vi "PH_Sequencer_Watch.ProcCases.vi"(0 "i ref in":refnum<vi>, 1 "selector":string, 2 "Data":T1, 3 "call cluster":T2={"Object"="", "Selector"="", "CallType"=enum."synchronous", "Async Object"="", "Async Selector"="", "Data Descriptor"="", "Data"=[], "Error #"=0, "Expire"=0}, 5 "error in (no error)":errorcluster) -> (14 "i ref out":refnum<vi>, 17 "answer cluster":T2={"Object"="", "Selector"="", "CallType"=enum."synchronous", "Async Object"="", "Async Selector"="", "Data Descriptor"="", "Data"=[], "Error #"=0, "Expire"=0}, 19 "error out":errorcluster)   [LabVIEW 2014, in "PH_Sequencer_Watch.lvlib"]
doc: "This method is called by a process from within the default case in the event loop. The methods of a class that are linked to events will be called from THIS method. Add your code here."
uses:
  PH_Sequencer_Watch.lvlib
  CSCore/CSSystem/CoreDefs/CoreDefs.call_type.ctl
  CSCore/BaseProcess/BaseProcess.descriptor string definition.ctl
  CSCore/CSSystem/CoreDefs/CoreDefs.rawDataType.ctl
  PH_PP_Common/PH_PP_Common.PUs.ctl
  CSCore/CSSystem/CoreLib/CoreLib.string 2 byte array.vi
  CSCore/BaseProcess/BaseProcess.lvlib
  CSCore/CAEObj/CAEObj.lvlib
  CSCore/CSSystem/CoreLib/CoreLib.lvlib
  PH_Common/PH_Common.lvlib
  lib.lib/DimLVEvent/LVDimInterface/LVDimInterface.lvlib
  PH_StatusHandler/PH_StatusHandler.lvlib
  PH_BeamlineInformation/PH_BeamlineInformation.lvlib
  PH_SystemInformation/PH_SystemInformation.lvlib
  PH_PP_Common/PH_PP_Common.lvlib
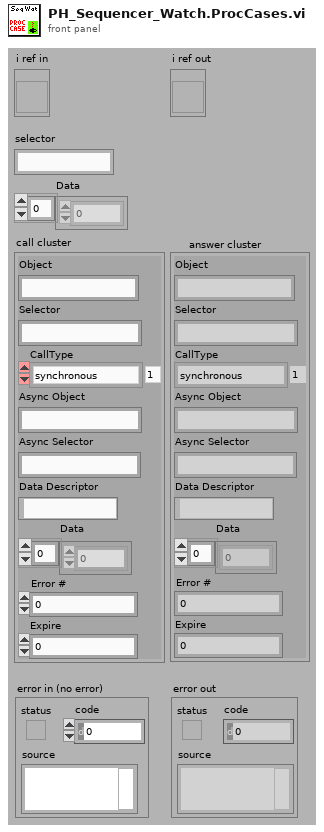
[diagram p1: front panel]
types:
  T1 = typedef "CoreDefs.rawDataType.ctl" = i8[]
  T2 = typedef "CoreDefs.call_type.ctl" = cluster{"Object":string, "Selector":string, "CallType":enum16{"simple", "synchronous", "asynchronous"}, "Async Object":string, "Async Selector":string, "Data Descriptor":T3, "Data":T1, "Error #":i32, "Expire":u32}
  T3 = typedef "BaseProcess.lvlib/BaseProcess.descriptor string definition.ctl" = string
  T4 = typedef "PH_Sequencer_Watch.lvlib/PH_Sequencer_Watch.i attribute.ctl" = cluster{"GUI Refs":cluster{"Shot ID":refnum<vi>, "Sequencer SM State":refnum<vi>, "Remaining Time":refnum<vi>, "PHELIX_Timing_T2":refnum<vi>, "T2-Unit-Dummy":refnum<vi>, "fs_Synchrolock_Watch":refnum<vi>, "Experiment_Vacuum_Control_Experiment":refnum<vi>}, "Status Synchrolock":T5, "Exp - Pressure":dbl, "Exp - Limit":dbl, "Heads":T6[], "Refs BooleanState":refnum<vi>[]}
  T5 = typedef "PH_StatusHandler.lvlib/PH_StatusHandler.Status.ctl" = i16
  T6 = typedef "PH_Sequencer_Watch.lvlib/PH_Sequencer_Watch.Head Information.ctl" = cluster{"Ref Volt":refnum<vi>, "PU":T7}
  T7 = typedef "PH_PP_Common.lvlib/PH_PP_Common.PUs.ctl" = enum16{"no Info", "PA-19mm-1", "PA-19mm-2", "PA-45mm-PILC", "PA-45mm-MAIN", "MA-PU-1", "MA-PU-2", "MA-PU-3", "MA-PU-4", "MA-PU-5", "MA-PU-6", "MA-FR", "MA-PILC", "PA-45mm-DP"}
  T8 = typedef "PH_BeamlineInformation.lvlib/PH_BeamlineInformation.i attribute.ctl" = cluster{"BL GUI Elements of Services":cluster{"Service Name":string, "GUI Elements":refnum<vi>[], "Status":i32}[], "Powermeters":T9, "Efficiency":T10, "Heads":T11[]}
  T9 = typedef "PH_BeamlineInformation.lvlib/PH_BeamlineInformation.Powermeter.ctl" = cluster{"ns FE":cluster{"GUI Ref":refnum<vi>, "Value":dbl}, "fs FE":cluster{"GUI Ref":refnum<vi>, "Value":dbl}, "PA":cluster{"GUI Ref":refnum<vi>, "Value":dbl}, "MA":cluster{"GUI Ref":refnum<vi>, "Value":dbl}, "Z6 green":cluster{"GUI Ref":refnum<vi>, "Value":dbl}, "Z6 IR":cluster{"GUI Ref":refnum<vi>, "Value":dbl}, "Z6 COS":cluster{"GUI Ref":refnum<vi>, "Value":dbl}}
  T10 = typedef "PH_BeamlineInformation.lvlib/PH_BeamlineInformation.Efficiency.ctl" = cluster{"PA Gain":cluster{"GUI Ref":refnum<vi>, "Value":dbl}, "MA Gain":cluster{"GUI Ref":refnum<vi>, "Value":dbl}, "Z6 green Conversion":cluster{"GUI Ref":refnum<vi>, "Value":dbl}, "Z6 Comp Losses":cluster{"GUI Ref":refnum<vi>, "Value":dbl}}
  T11 = typedef "PH_BeamlineInformation.lvlib/PH_BeamlineInformation.Head.ctl" = cluster{"PowerUnit":T7, "in use":cluster{"Value":bool, "GUI Ref":refnum<vi>, "linked":bool}, "voltage":cluster{"Value":dbl, "GUI Ref":refnum<vi>, "linked":bool}}
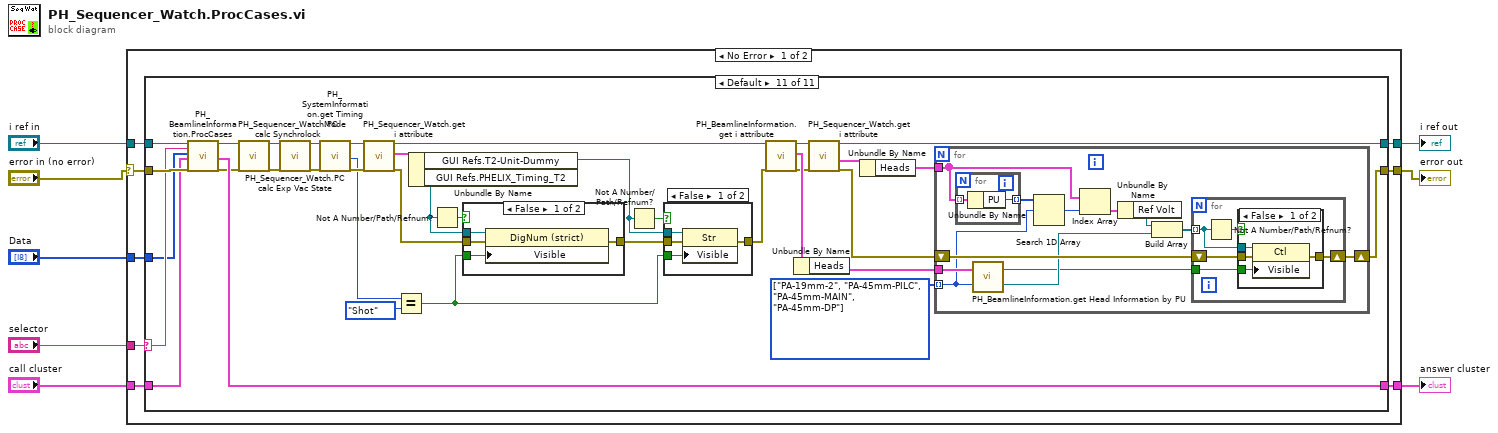
[diagram p0: block diagram]
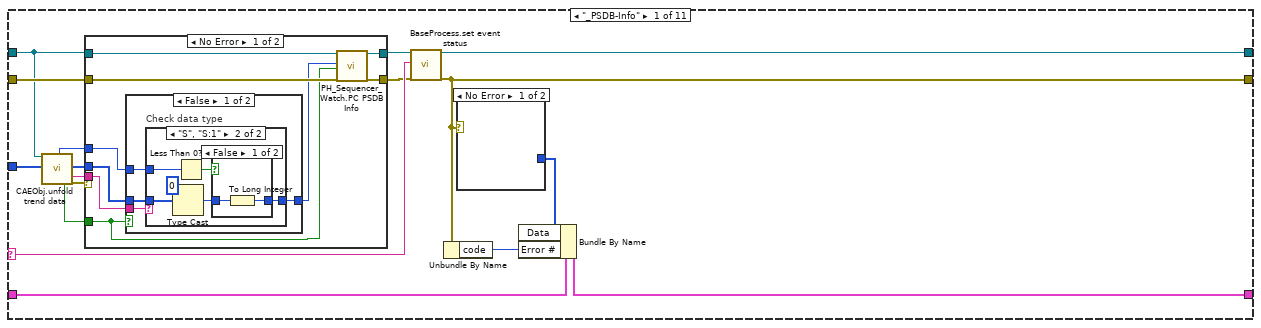
[diagram p2: hidden frame]
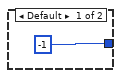
[diagram p3: hidden frame]
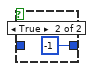
[diagram p4: hidden frame]
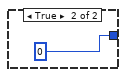
[diagram p5: hidden frame]
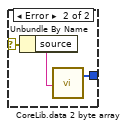
[diagram p7: hidden frame]
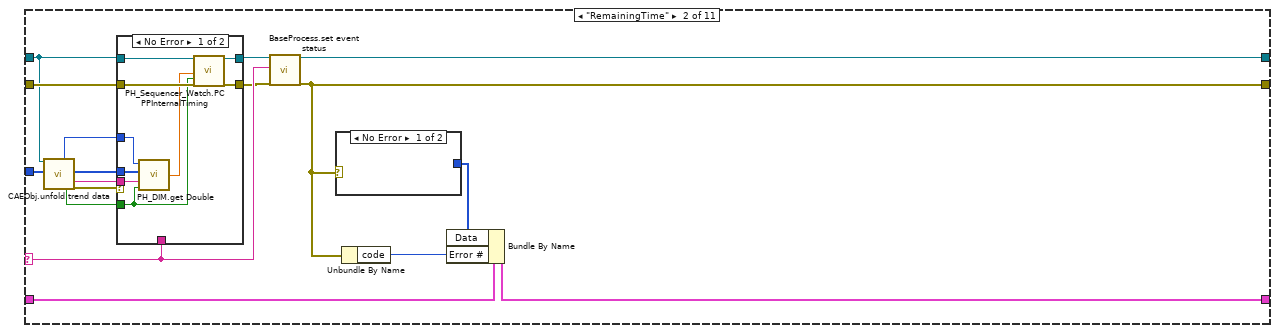
[diagram p8: hidden frame]
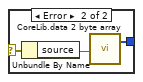
[diagram p9: hidden frame]
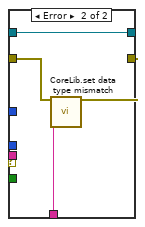
[diagram p10: hidden frame]
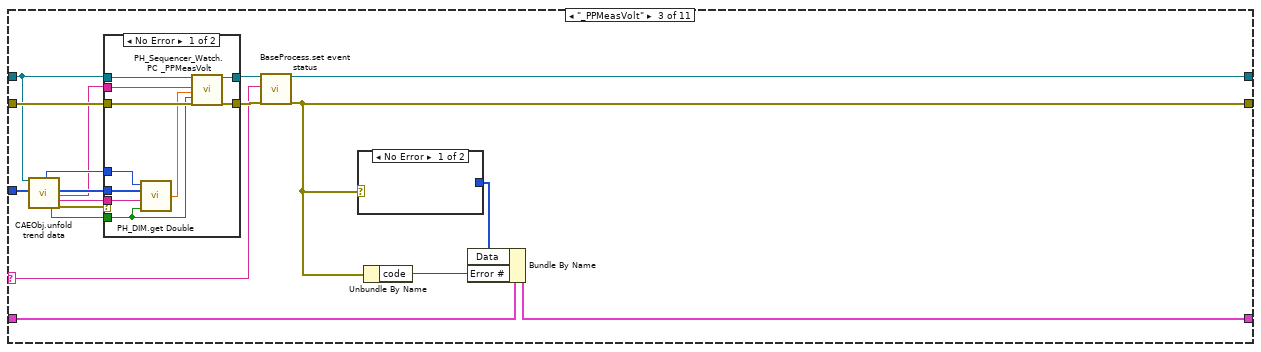
[diagram p11: hidden frame]
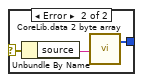
[diagram p12: hidden frame]
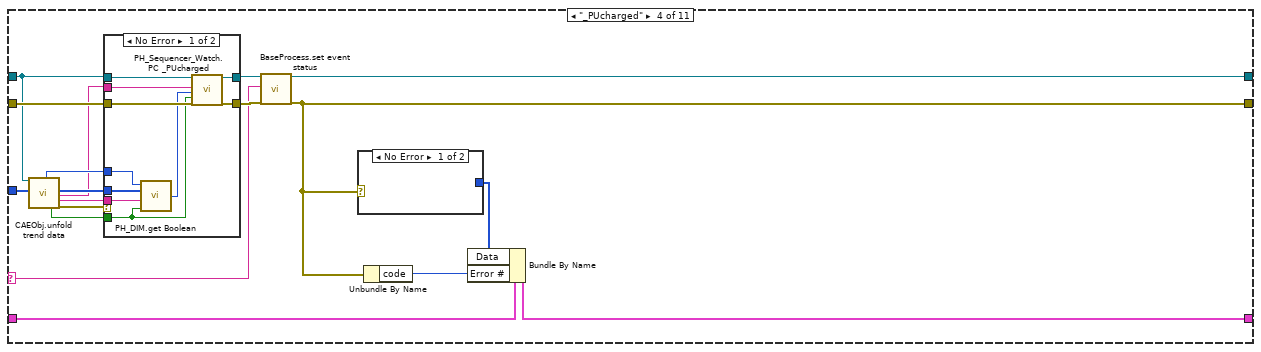
[diagram p14: hidden frame]
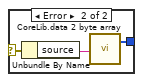
[diagram p15: hidden frame]
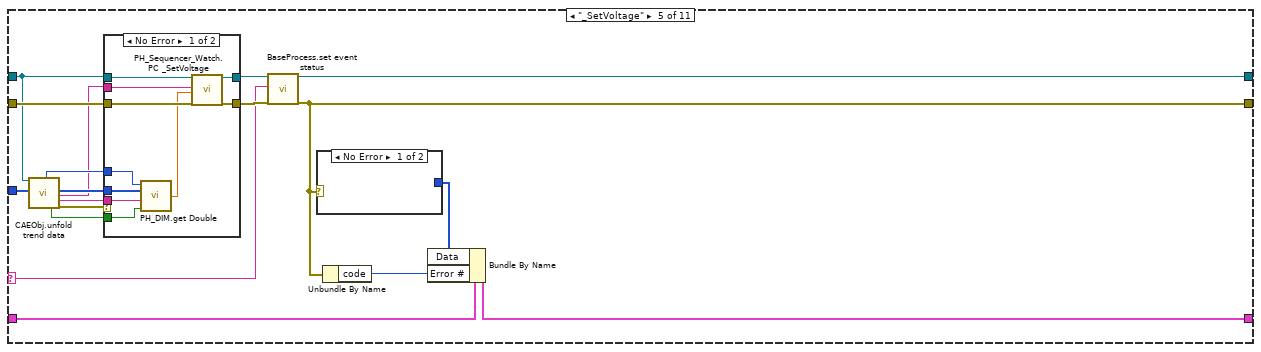
[diagram p17: hidden frame]
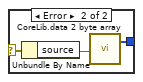
[diagram p18: hidden frame]
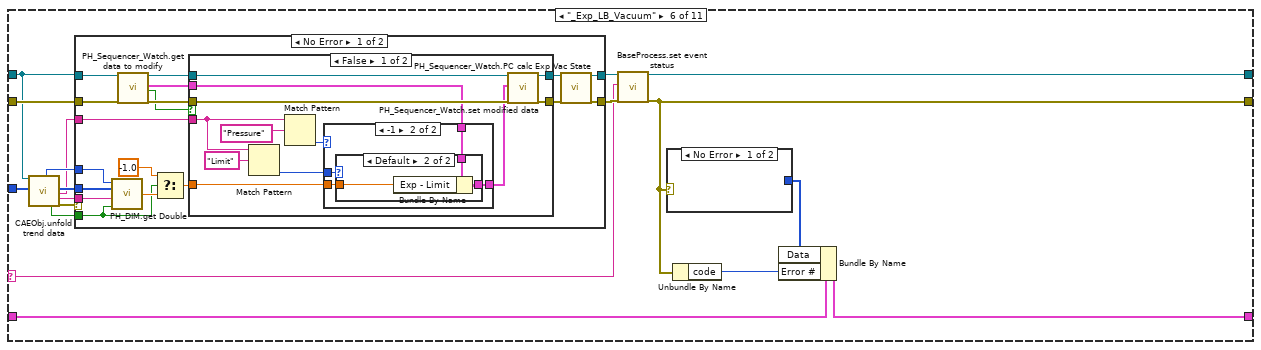
[diagram p20: hidden frame]
diagram:
  n1 = case shown="No Error" "error in (no error)" {
    selector: "error in (no error)" -> [w9 w474]
    tunnel: "selector" -> [w16 _]
    tunnel: [w15 w472] -> w7
    tunnel: "call cluster" -> [w14 w472]
    tunnel: "i ref in" -> [w13 w473]
    tunnel: [w12 w473] -> w4
    tunnel: [w11 w474] -> w3
    tunnel: "Data" -> [w10 _]
    frame No Error {
      n2 = case shown="Default" w16 {
        selector: w16 -> [w27 w76 w98 w131 w164 w197 w270 w308 w338 w381 w434]
        tunnel: w13 -> [w23 w68 w112 w145 w178 w211 w266 w304 w334 w378 w433]
        tunnel: [w31 w73 w99 w132 w165 w198 w272 w310 w340 w383 w409] -> w12
        tunnel: w14 -> [w28 w70 w97 w130 w163 w196 w268 w306 w336 w379 w435]
        tunnel: [w29 w71 w96 w129 w162 w195 w269 w307 w337 w380 w436] -> w15
        tunnel: w9 -> [w24 w79 w113 w146 w179 w212 w277 w302 w332 w376 w437]
        tunnel: [w30 w72 w100 w133 w166 w199 w271 w309 w339 w382 w410] -> w11
        tunnel: w10 -> [w22 w69 w111 w144 w177 w210 w267 w305 w335 w374 w432]
        frame "_PSDB-Info" {
          n3 = call "CAEObj.unfold trend data.vi"("i ref in"=w23, "raw trend data"=w22) -> ("quality"=w20:i32, "no link"=w19:bool, "data"=w17:i8[], "typeDescriptor"=w18:string, "error out"=w21:errorcluster)  [unwired: 9 in, 4 out]
          n4 = case shown="No Error" w21 {
            tunnel: [w40 w59] -> w26
            tunnel: [w39 w58] -> w25
            tunnel: w24 -> [w42 w58]
            tunnel: w23 -> [w41 w59]
            tunnel: w20 -> [w38 _]
            tunnel: w19 -> [w34 _]
            tunnel: w18 -> [w37 _]
            tunnel: w17 -> [w36 _]
            frame No Error {
              n5 = case "No link?" shown="False" w34 {
                tunnel: [w46 0] -> w35
                tunnel: w38 -> [w45 _]
                tunnel: w36 -> [w44 _]
                tunnel: w37 -> [w43 _]
                frame False {
                  n6 = case "Check data type" shown="\"S\", \"S:1\"" w43 {
                    tunnel: [-1 w53] -> w46
                    tunnel: w45 -> [_ w51]
                    tunnel: w44 -> [_ w49]
                    frame Default {
                    }
                    frame "S", "S:1" {
                      n7 = Type Cast(type=i16 0, x=w49) -> (*(type *) &x=w48:i16)
                      n8 = Less Than 0?(x=w51) -> (x < 0?=w52:bool)
                      n9 = case shown="False" w52 {
                        tunnel: [w54 -1] -> w53
                        tunnel: w48 -> [w55 _]
                        frame False {
                          n10 = To Long Integer(number=w55) -> (32bit integer=w54:i32)
                        }
                        frame True {
                        }
                      }
                    }
                  }
                }
                frame True {
                }
              }
              n11 = call "PH_Sequencer_Watch.PC PSDB Info.vi"("i ref in"=w41, "Shot ID"=w35, "no link?"=w34, "error IO"=w42) -> ("i ref out"=w40:refnum<vi>, "error out"=w39:errorcluster)  [unwired: 14 in]
            }
            frame Error {
            }
          }
          n12 = call "BaseProcess.set event status.vi"("i ref in"=w26, "EventStatus"=w27, "error in (no error)"=w25) -> ("i ref out"=w31:refnum<vi>, "error out"=w30:errorcluster)  [unwired: 14 in, 1 out]
          n13 = Unbundle By Name(w30) -> ("code"=w33:i32)
          n14 = case shown="No Error" w30 {
            selector: w30 -> [_ w62]
            tunnel: [_ w60] -> w32
            frame No Error {
            }
            frame Error {
              n15 = Unbundle By Name(w62) -> ("source"=w61:string)
              n16 = call-poly "CoreLib.data 2 byte array.vi"("string"=w61) -> ("byteArray out"=w60:T1)  [unwired: 18 in]
            }
          }
          n17 = Bundle By Name(cluster=w28, "Data"=w32, "Error #"=w33) -> (w29:T2)
        }
        frame "RemainingTime" {
          n18 = call "CAEObj.unfold trend data.vi"("i ref in"=w68, "raw trend data"=w69) -> ("quality"=w64:i32, "no link"=w66:bool, "data"=w65:i8[], "typeDescriptor"=w63:string, "error out"=w67:errorcluster)  [unwired: 9 in, 4 out]
          n19 = case shown="No Error" w67 {
            tunnel: [w89 w95] -> w75
            tunnel: w68 -> [w91 w95]
            tunnel: w79 -> [w90 w94]
            tunnel: [w88 w93] -> w74
            tunnel: w76 -> [_ w92]
            tunnel: w66 -> [w84 _]
            tunnel: w65 -> [w87 _]
            tunnel: w64 -> [w86 _]
            tunnel: w63 -> [w85 _]
            frame No Error {
              n20 = call "PH_DIM.get Double.vi"("no link"=w84, "typeDescriptor"=w85, "data"=w87, "quality"=w86) -> ("Value"=w83:dbl)
              n21 = call "PH_Sequencer_Watch.PC PPInternalTiming.vi"("i ref in"=w91, "Remaining Time [s]"=w83, "no link?"=w84, "error in (no error)"=w90) -> ("i ref out"=w89:refnum<vi>, "error out"=w88:errorcluster)  [unwired: 14 in]
            }
            frame Error {
              n22 = call "CoreLib.set data type mismatch.vi"("error in (no error)"=w94, "error source"=w92) -> ("error out"=w93:errorcluster)  [unwired: 17 in]
            }
          }
          n23 = call "BaseProcess.set event status.vi"("i ref in"=w75, "EventStatus"=w76, "error in (no error)"=w74) -> ("i ref out"=w73:refnum<vi>, "error out"=w72:errorcluster)  [unwired: 14 in, 1 out]
          n24 = case shown="No Error" w72 {
            selector: w72 -> [_ w82]
            tunnel: [_ w80] -> w77
            frame No Error {
            }
            frame Error {
              n25 = Unbundle By Name(w82) -> ("source"=w81:string)
              n26 = call-poly "CoreLib.data 2 byte array.vi"("string"=w81) -> ("byteArray out"=w80:T1)  [unwired: 18 in]
            }
          }
          n27 = Unbundle By Name(w72) -> ("code"=w78:i32)
          n28 = Bundle By Name(cluster=w70, "Data"=w77, "Error #"=w78) -> (w71:T2)
        }
        frame "_PPMeasVolt" {
          n29 = call "CAEObj.unfold trend data.vi"("i ref in"=w112, "raw trend data"=w111) -> ("quality"=w107:i32, "no link"=w106:bool, "data"=w108:i8[], "serviceName"=w105:string, "typeDescriptor"=w109:string, "error out"=w110:errorcluster)  [unwired: 9 in, 3 out]
          n30 = case shown="No Error" w110 {
            tunnel: [w124 w128] -> w101
            tunnel: w112 -> [w126 w128]
            tunnel: w113 -> [w125 w127]
            tunnel: [w123 w127] -> w102
            tunnel: w109 -> [w122 _]
            tunnel: w108 -> [w121 _]
            tunnel: w107 -> [w120 _]
            tunnel: w106 -> [w117 _]
            tunnel: w105 -> [w118 _]
            frame No Error {
              n31 = call "PH_DIM.get Double.vi"("no link"=w117, "typeDescriptor"=w122, "data"=w121, "quality"=w120) -> ("Value"=w119:dbl)
              n32 = call "PH_Sequencer_Watch.PC _PPMeasVolt.vi"("i ref in"=w126, "Tagname"=w118, "Tagvalue"=w119, "no link"=w117, "error in (no error)"=w125) -> ("i ref out"=w124:refnum<vi>, "error out"=w123:errorcluster)  [unwired: 13 in]
            }
            frame Error {
            }
          }
          n33 = call "BaseProcess.set event status.vi"("i ref in"=w101, "EventStatus"=w98, "error in (no error)"=w102) -> ("i ref out"=w99:refnum<vi>, "error out"=w100:errorcluster)  [unwired: 14 in, 1 out]
          n34 = case shown="No Error" w100 {
            selector: w100 -> [_ w116]
            tunnel: [_ w114] -> w103
            frame No Error {
            }
            frame Error {
              n35 = Unbundle By Name(w116) -> ("source"=w115:string)
              n36 = call-poly "CoreLib.data 2 byte array.vi"("string"=w115) -> ("byteArray out"=w114:T1)  [unwired: 18 in]
            }
          }
          n37 = Unbundle By Name(w100) -> ("code"=w104:i32)
          n38 = Bundle By Name(cluster=w97, "Data"=w103, "Error #"=w104) -> (w96:T2)
        }
        frame "_PUcharged" {
          n39 = call "CAEObj.unfold trend data.vi"("i ref in"=w145, "raw trend data"=w144) -> ("quality"=w140:i32, "no link"=w139:bool, "data"=w141:i8[], "serviceName"=w138:string, "typeDescriptor"=w142:string, "error out"=w143:errorcluster)  [unwired: 9 in, 3 out]
          n40 = case shown="No Error" w143 {
            tunnel: [w157 w161] -> w134
            tunnel: w145 -> [w159 w161]
            tunnel: w146 -> [w158 w160]
            tunnel: [w156 w160] -> w135
            tunnel: w142 -> [w155 _]
            tunnel: w141 -> [w154 _]
            tunnel: w140 -> [w153 _]
            tunnel: w139 -> [w150 _]
            tunnel: w138 -> [w151 _]
            frame No Error {
              n41 = call "PH_DIM.get Boolean.vi"("no link"=w150, "typeDescriptor"=w155, "data"=w154, "quality"=w153) -> ("Value"=w152:i32)
              n42 = call "PH_Sequencer_Watch.PC _PUcharged.vi"("i ref in"=w159, "Tagname"=w151, "Tagvalue"=w152, "no link"=w150, "error in (no error)"=w158) -> ("i ref out"=w157:refnum<vi>, "error out"=w156:errorcluster)  [unwired: 13 in]
            }
            frame Error {
            }
          }
          n43 = call "BaseProcess.set event status.vi"("i ref in"=w134, "EventStatus"=w131, "error in (no error)"=w135) -> ("i ref out"=w132:refnum<vi>, "error out"=w133:errorcluster)  [unwired: 14 in, 1 out]
          n44 = case shown="No Error" w133 {
            selector: w133 -> [_ w149]
            tunnel: [_ w147] -> w136
            frame No Error {
            }
            frame Error {
              n45 = Unbundle By Name(w149) -> ("source"=w148:string)
              n46 = call-poly "CoreLib.data 2 byte array.vi"("string"=w148) -> ("byteArray out"=w147:T1)  [unwired: 18 in]
            }
          }
          n47 = Unbundle By Name(w133) -> ("code"=w137:i32)
          n48 = Bundle By Name(cluster=w130, "Data"=w136, "Error #"=w137) -> (w129:T2)
        }
        frame "_SetVoltage" {
          n49 = call "CAEObj.unfold trend data.vi"("i ref in"=w178, "raw trend data"=w177) -> ("quality"=w173:i32, "no link"=w172:bool, "data"=w174:i8[], "serviceName"=w171:string, "typeDescriptor"=w175:string, "error out"=w176:errorcluster)  [unwired: 9 in, 3 out]
          n50 = case shown="No Error" w176 {
            tunnel: [w190 w194] -> w167
            tunnel: w178 -> [w192 w194]
            tunnel: w179 -> [w191 w193]
            tunnel: [w189 w193] -> w168
            tunnel: w175 -> [w188 _]
            tunnel: w174 -> [w187 _]
            tunnel: w173 -> [w186 _]
            tunnel: w172 -> [w183 _]
            tunnel: w171 -> [w184 _]
            frame No Error {
              n51 = call "PH_DIM.get Double.vi"("no link"=w183, "typeDescriptor"=w188, "data"=w187, "quality"=w186) -> ("Value"=w185:dbl)
              n52 = call "PH_Sequencer_Watch.PC _SetVoltage.vi"("i ref in"=w192, "Tagname"=w184, "Tagvalue"=w185, "error in (no error)"=w191) -> ("i ref out"=w190:refnum<vi>, "error out"=w189:errorcluster)  [unwired: 14 in]
            }
            frame Error {
            }
          }
          n53 = call "BaseProcess.set event status.vi"("i ref in"=w167, "EventStatus"=w164, "error in (no error)"=w168) -> ("i ref out"=w165:refnum<vi>, "error out"=w166:errorcluster)  [unwired: 14 in, 1 out]
          n54 = case shown="No Error" w166 {
            selector: w166 -> [_ w182]
            tunnel: [_ w180] -> w169
            frame No Error {
            }
            frame Error {
              n55 = Unbundle By Name(w182) -> ("source"=w181:string)
              n56 = call-poly "CoreLib.data 2 byte array.vi"("string"=w181) -> ("byteArray out"=w180:T1)  [unwired: 18 in]
            }
          }
          n57 = Unbundle By Name(w166) -> ("code"=w170:i32)
          n58 = Bundle By Name(cluster=w163, "Data"=w169, "Error #"=w170) -> (w162:T2)
        }
        frame "_Exp_LB_Vacuum" {
          n59 = call "CAEObj.unfold trend data.vi"("i ref in"=w211, "raw trend data"=w210) -> ("quality"=w206:i32, "no link"=w205:bool, "data"=w207:i8[], "serviceName"=w204:string, "typeDescriptor"=w208:string, "error out"=w209:errorcluster)  [unwired: 9 in, 3 out]
          n60 = case shown="No Error" w209 {
            tunnel: [w226 w260] -> w200
            tunnel: w211 -> [w233 w260]
            tunnel: w212 -> [w232 w259]
            tunnel: [w227 w259] -> w201
            tunnel: w208 -> [w230 _]
            tunnel: w207 -> [w229 _]
            tunnel: w206 -> [w228 _]
            tunnel: w205 -> [w218 _]
            tunnel: w204 -> [w221 _]
            frame No Error {
              n61 = call "PH_DIM.get Double.vi"("no link"=w218, "typeDescriptor"=w230, "data"=w229, "quality"=w228) -> ("Value"=w219:dbl)
              n62 = call "PH_Sequencer_Watch.get data to modify.vi"("i ref in"=w233, "error in (no error)"=w232) -> ("i ref out"=w224:refnum<vi>, "i attribute"=w220:T4, "timed out"=w222:bool, "error out"=w231:errorcluster)  [unwired: 14 in]
              n63 = Select(t=-1.0, s=w218, f=w219) -> (s? t:f=w216:dbl)
              n64 = case shown="False" w222 {
                tunnel: w231 -> [w245 w257]
                tunnel: [w244 w257] -> w225
                tunnel: w224 -> [w243 w258]
                tunnel: [w242 w258] -> w223
                tunnel: w221 -> [w236 _]
                tunnel: w220 -> [w240 _]
                tunnel: w216 -> [w237 _]
                frame False {
                  n65 = Match Pattern(string=w236, regular expression="Limit") -> (offset past match=w234:i32)  [unwired: 1 in, 3 out]
                  n66 = Match Pattern(string=w236, regular expression="Pressure") -> (offset past match=w239:i32)  [unwired: 1 in, 3 out]
                  n67 = case shown="-1" w239 {
                    tunnel: w240 -> [w248 w252]
                    tunnel: [w247 w251] -> w238
                    tunnel: w237 -> [w246 w250]
                    tunnel: w234 -> [_ w249]
                    frame Default {
                      n68 = Bundle By Name(cluster=w248, "Exp - Pressure"=w246) -> (w247:T4)
                    }
                    frame -1 {
                      n69 = case shown="Default" w249 {
                        tunnel: w252 -> [w253 w256]
                        tunnel: [w253 w255] -> w251
                        tunnel: w250 -> [_ w254]
                        frame 0 {
                        }
                        frame Default {
                          n70 = Bundle By Name(cluster=w256, "Exp - Limit"=w254) -> (w255:T4)
                        }
                      }
                    }
                  }
                  n71 = call "PH_Sequencer_Watch.set modified data.vi"("i ref in"=w243, "i attribute"=w238, "error in (no error)"=w245) -> ("i ref out"=w242:refnum<vi>, "error out"=w244:errorcluster)  [unwired: 15 in]
                }
                frame True {
                }
              }
              n72 = call "PH_Sequencer_Watch.PC calc Exp Vac State.vi"("i ref in"=w223, "error in"=w225) -> ("i ref out"=w226:refnum<vi>, "error out"=w227:errorcluster)  [unwired: 16 in]
            }
            frame Error {
            }
          }
          n73 = call "BaseProcess.set event status.vi"("i ref in"=w200, "EventStatus"=w197, "error in (no error)"=w201) -> ("i ref out"=w198:refnum<vi>, "error out"=w199:errorcluster)  [unwired: 14 in, 1 out]
          n74 = case shown="No Error" w199 {
            selector: w199 -> [_ w215]
            tunnel: [_ w213] -> w202
            frame No Error {
            }
            frame Error {
              n75 = Unbundle By Name(w215) -> ("source"=w214:string)
              n76 = call-poly "CoreLib.data 2 byte array.vi"("string"=w214) -> ("byteArray out"=w213:T1)  [unwired: 18 in]
            }
          }
          n77 = Unbundle By Name(w199) -> ("code"=w203:i32)
          n78 = Bundle By Name(cluster=w196, "Data"=w202, "Error #"=w203) -> (w195:T2)
        }
        frame "_Sequencer_SM_State" {
          n79 = call "CAEObj.unfold trend data.vi"("i ref in"=w266, "raw trend data"=w267) -> ("quality"=w261:i32, "no link"=w262:bool, "data"=w264:i8[], "typeDescriptor"=w263:string, "error out"=w265:errorcluster)  [unwired: 9 in, 4 out]
          n80 = case shown="No Error" w265 {
            tunnel: [w287 w295] -> w273
            tunnel: w266 -> [w288 w295]
            tunnel: w277 -> [w290 w294]
            tunnel: [w285 w294] -> w274
            tunnel: w264 -> [w293 _]
            tunnel: w263 -> [w292 _]
            tunnel: w262 -> [w283 _]
            tunnel: w261 -> [w291 _]
            frame No Error {
              n81 = call "PH_Sequencer_Watch.get i attribute.vi"("i ref in"=w288, "error in (no error)"=w290) -> ("i ref out"=w287:refnum<vi>, "i attribute"=w286:T4, "error out"=w289:errorcluster)  [unwired: 15 in]
              n82 = call "PH_DIM.get String.vi"("no link"=w283, "typeDescriptor"=w292, "data"=w293, "quality"=w291) -> ("Output String"=w282:string)
              n83 = Unbundle By Name(w286) -> ("GUI Refs.Sequencer SM State"=w284:refnum<vi>)
              n84 = call "PH_Strings.Remove trailing Zeros.vi"("Input String"=w282) -> ("Output String"=w281:string)
              n85 = call "PH_GUI.set string GUI object.vi"("GUI object Ref"=w284, "Text"=w281, "Blinking? (false)"=w283, "error in"=w289) -> ("error out"=w285:errorcluster)  [unwired: 15 in]
            }
            frame Error {
            }
          }
          n86 = call "BaseProcess.set event status.vi"("i ref in"=w273, "EventStatus"=w270, "error in (no error)"=w274) -> ("i ref out"=w272:refnum<vi>, "error out"=w271:errorcluster)  [unwired: 14 in, 1 out]
          n87 = case shown="No Error" w271 {
            selector: w271 -> [_ w280]
            tunnel: [_ w278] -> w275
            frame No Error {
            }
            frame Error {
              n88 = Unbundle By Name(w280) -> ("source"=w279:string)
              n89 = call-poly "CoreLib.data 2 byte array.vi"("string"=w279) -> ("byteArray out"=w278:T1)  [unwired: 18 in]
            }
          }
          n90 = Unbundle By Name(w271) -> ("code"=w276:i32)
          n91 = Bundle By Name(cluster=w268, "Data"=w275, "Error #"=w276) -> (w269:T2)
        }
        frame "_BoleanStates" {
          n92 = call "CAEObj.unfold trend data.vi"("i ref in"=w304, "raw trend data"=w305) -> ("no link"=w297:bool, "data"=w300:i8[], "serviceName"=w296:string, "typeDescriptor"=w298:string, "error out"=w299:errorcluster)  [unwired: 9 in, 4 out]
          n93 = case shown="No Error" w299 {
            tunnel: [w318 w323] -> w303
            tunnel: w304 -> [w319 w323]
            tunnel: w302 -> [w321 w322]
            tunnel: [w320 w322] -> w301
            tunnel: w297 -> [w314 _]
            tunnel: w300 -> [w316 _]
            tunnel: w298 -> [w315 _]
            tunnel: w296 -> [w317 _]
            frame No Error {
              n94 = call "PH_StatusHandler.get Status DIM Service.vi"("no link"=w314, "typeDescriptor"=w315, "data"=w316) -> ("Status"=w313:T5)  [unwired: 1 in]
              n95 = call "PH_Sequencer_Watch.PC _BooleanState.vi"("i ref in"=w319, "serviceName"=w317, "Status"=w313, "error IO"=w321) -> ("i ref out"=w318:refnum<vi>, "error out"=w320:errorcluster)  [unwired: 14 in]
            }
            frame Error {
            }
          }
          n96 = call "BaseProcess.set event status.vi"("i ref in"=w303, "EventStatus"=w308, "error in (no error)"=w301) -> ("i ref out"=w310:refnum<vi>, "error out"=w309:errorcluster)  [unwired: 14 in, 1 out]
          n97 = case shown="No Error" w309 {
            selector: w309 -> [_ w326]
            tunnel: [_ w324] -> w311
            frame No Error {
            }
            frame Error {
              n98 = Unbundle By Name(w326) -> ("source"=w325:string)
              n99 = call-poly "CoreLib.data 2 byte array.vi"("string"=w325) -> ("byteArray out"=w324:T1)  [unwired: 18 in]
            }
          }
          n100 = Unbundle By Name(w309) -> ("code"=w312:i32)
          n101 = Bundle By Name(cluster=w306, "Data"=w311, "Error #"=w312) -> (w307:T2)
        }
        frame "_fs_Synchrolock" {
          n102 = call "CAEObj.unfold trend data.vi"("i ref in"=w334, "raw trend data"=w335) -> ("no link"=w327:bool, "data"=w330:i8[], "typeDescriptor"=w328:string, "error out"=w329:errorcluster)  [unwired: 9 in, 5 out]
          n103 = case shown="No Error" w329 {
            tunnel: [w346 w367] -> w333
            tunnel: w334 -> [w354 w367]
            tunnel: w332 -> [w356 w366]
            tunnel: [w349 w366] -> w331
            tunnel: w327 -> [w351 _]
            tunnel: w330 -> [w353 _]
            tunnel: w328 -> [w352 _]
            frame No Error {
              n104 = call "PH_StatusHandler.get Status DIM Service.vi"("no link"=w351, "typeDescriptor"=w352, "data"=w353) -> ("Status"=w343:T5)  [unwired: 1 in]
              n105 = call "PH_Sequencer_Watch.get data to modify.vi"("i ref in"=w354, "error in (no error)"=w356) -> ("i ref out"=w348:refnum<vi>, "i attribute"=w344:T4, "timed out"=w345:bool, "error out"=w355:errorcluster)  [unwired: 14 in]
              n106 = case shown="False" w345 {
                tunnel: w355 -> [w363 w364]
                tunnel: [w362 w364] -> w350
                tunnel: w348 -> [w361 w365]
                tunnel: [w360 w365] -> w347
                tunnel: w344 -> [w359 _]
                tunnel: w343 -> [w357 _]
                frame False {
                  n107 = Bundle By Name(cluster=w359, "Status Synchrolock"=w357) -> (w358:T4)
                  n108 = call "PH_Sequencer_Watch.set modified data.vi"("i ref in"=w361, "i attribute"=w358, "error in (no error)"=w363) -> ("i ref out"=w360:refnum<vi>, "error out"=w362:errorcluster)  [unwired: 15 in]
                }
                frame True {
                }
              }
              n109 = call "PH_Sequencer_Watch.PC calc Synchrolock.vi"("i ref in"=w347, "error in"=w350) -> ("i ref out"=w346:refnum<vi>, "error out"=w349:errorcluster)  [unwired: 16 in]
            }
            frame Error {
            }
          }
          n110 = call "BaseProcess.set event status.vi"("i ref in"=w333, "EventStatus"=w338, "error in (no error)"=w331) -> ("i ref out"=w340:refnum<vi>, "error out"=w339:errorcluster)  [unwired: 14 in, 1 out]
          n111 = case shown="No Error" w339 {
            selector: w339 -> [_ w370]
            tunnel: [_ w368] -> w341
            frame No Error {
            }
            frame Error {
              n112 = Unbundle By Name(w370) -> ("source"=w369:string)
              n113 = call-poly "CoreLib.data 2 byte array.vi"("string"=w369) -> ("byteArray out"=w368:T1)  [unwired: 18 in]
            }
          }
          n114 = Unbundle By Name(w339) -> ("code"=w342:i32)
          n115 = Bundle By Name(cluster=w336, "Data"=w341, "Error #"=w342) -> (w337:T2)
        }
        frame "_T2" {
          n116 = call "LVDimInterface.dim_unfold_data.vi"("rawData"=w374) -> ("data"=w372:i8[], "no link"=w371:bool, "error out"=w373:errorcluster)  [unwired: 15 in, 1 out]
          n117 = case shown="No Error" w373 {
            tunnel: [w390 w398] -> w377
            tunnel: w378 -> [w394 w398]
            tunnel: w376 -> [w393 w397]
            tunnel: [w387 w397] -> w375
            tunnel: w372 -> [w395 _]
            tunnel: w371 -> [w386 _]
            frame No Error {
              n118 = call "PH_Sequencer_Watch.get i attribute.vi"("i ref in"=w394, "error in (no error)"=w393) -> ("i ref out"=w390:refnum<vi>, "i attribute"=w392:T4, "error out"=w391:errorcluster)  [unwired: 15 in]
              n119 = Type Cast(type=i16 0, x=w395) -> (*(type *) &x=w388:i16)
              n120 = Unbundle By Name(w392) -> ("GUI Refs.PHELIX_Timing_T2"=w389:refnum<vi>)
              n121 = call "PH_GUI.set I16 GUI object.vi"("I16 GUI Ref"=w389, "value"=w388, "blinking (false)"=w386, "error in (no error)"=w391) -> ("error out"=w387:errorcluster)  [unwired: 15 in]
            }
            frame Error {
            }
          }
          n122 = call "BaseProcess.set event status.vi"("i ref in"=w377, "EventStatus"=w381, "error in (no error)"=w375) -> ("i ref out"=w383:refnum<vi>, "error out"=w382:errorcluster)  [unwired: 14 in, 1 out]
          n123 = case shown="No Error" w382 {
            selector: w382 -> [_ w401]
            tunnel: [_ w399] -> w384
            frame No Error {
            }
            frame Error {
              n124 = Unbundle By Name(w401) -> ("source"=w400:string)
              n125 = call-poly "CoreLib.data 2 byte array.vi"("string"=w400) -> ("byteArray out"=w399:T1)  [unwired: 18 in]
            }
          }
          n126 = Unbundle By Name(w382) -> ("code"=w385:i32)
          n127 = Bundle By Name(cluster=w379, "Data"=w384, "Error #"=w385) -> (w380:T2)
        }
        frame Default {
          w403 = T7[] [enum."PA-19mm-2", enum."PA-45mm-PILC", enum."PA-45mm-MAIN", enum."PA-45mm-DP"] items=["no Info", "PA-19mm-1", "PA-19mm-2", "PA-45mm-PILC", "PA-45mm-MAIN", "MA-PU-1", "MA-PU-2", "MA-PU-3", "MA-PU-4", "MA-PU-5", "MA-PU-6", "MA-FR", "MA-PILC", "PA-45mm-DP"]
          # "In the default case, always call the ProcCase method of the parent class"
          n128 = call "PH_BeamlineInformation.ProcCases.vi"("i ref in"=w433, "selector"=w434, "Data"=w432, "call cluster"=w435, "error in (no error)"=w437) -> ("i ref out"=w416:refnum<vi>, "answer cluster"=w436:T2, "error out"=w418:errorcluster)  [unwired: 12 in]
          n129 = call "PH_Sequencer_Watch.PC calc Synchrolock.vi"("i ref in"=w416, "error in"=w418) -> ("i ref out"=w417:refnum<vi>, "error out"=w419:errorcluster)  [unwired: 16 in]
          n130 = call "PH_Sequencer_Watch.PC calc Exp Vac State.vi"("i ref in"=w417, "error in"=w419) -> ("i ref out"=w415:refnum<vi>, "error out"=w414:errorcluster)  [unwired: 16 in]
          n131 = call "PH_SystemInformation.get Timing Mode.vi"("i ref in"=w415, "error in (no error)"=w414) -> ("i ref out"=w427:refnum<vi>, "PHELIX Timing Mode"=w430:enum32{"10 Hz", "0.5 Hz", "Shot"}, "error out"=w431:errorcluster)  [unwired: 15 in]
          n132 = call "PH_Sequencer_Watch.get i attribute.vi"("i ref in"=w427, "error in (no error)"=w431) -> ("i ref out"=w412:refnum<vi>, "i attribute"=w426:T4, "error out"=w428:errorcluster)  [unwired: 15 in]
          n133 = Equal?(x=w430, y=enum32{"10 Hz", "0.5 Hz", "Shot"}."Shot") -> (x = y?=w420:bool)
          n134 = Unbundle By Name(w426) -> ("GUI Refs.T2-Unit-Dummy"=w421:refnum<vi>, "GUI Refs.PHELIX_Timing_T2"=w425:refnum<vi>)
          n135 = Not A Number/Path/Refnum?(number/path/refnum=w425) -> (NaN/Path/Refnum?=w424:bool)
          n136 = case shown="False" w424 {
            tunnel: w428 -> [w470 w471]
            tunnel: [w469 w471] -> w422
            tunnel: w425 -> [w468 _]
            tunnel: w420 -> [w467 _]
            frame False {
              n137 = property class="DigNum (strict)"(reference=w468, error in=w470, "Visible"=w467) -> (error out=w469:errorcluster)  [unwired: 1 out]
            }
            frame True {
            }
          }
          n138 = Not A Number/Path/Refnum?(number/path/refnum=w421) -> (NaN/Path/Refnum?=w423:bool)
          n139 = case shown="False" w423 {
            tunnel: w422 -> [w465 w466]
            tunnel: [w464 w466] -> w406
            tunnel: w421 -> [w463 _]
            tunnel: w420 -> [w462 _]
            frame False {
              n140 = property class="Str"(reference=w463, error in=w465, "Visible"=w462) -> (error out=w464:errorcluster)  [unwired: 1 out]
            }
            frame True {
            }
          }
          n141 = call "PH_BeamlineInformation.get i attribute.vi"("i ref in"=w412, "error in (no error)"=w406) -> ("i ref out"=w411:refnum<vi>, "i attribute"=w413:T8, "error out"=w408:errorcluster)  [unwired: 15 in]
          n142 = Unbundle By Name(w413) -> ("Heads"=w402:T11[])
          n143 = call "PH_Sequencer_Watch.get i attribute.vi"("i ref in"=w411, "error in (no error)"=w408) -> ("i ref out"=w409:refnum<vi>, "i attribute"=w405:T4, "error out"=w407:errorcluster)  [unwired: 15 in]
          n144 = Unbundle By Name(w405) -> ("Heads"=w404:T6[])
          n145 = for {
            tunnel: w403 -> [w438] mode=indexing
            tunnel: w404 -> [w442]
            shift-right: [w449] -> w410
            shift-left: w407 -> [w448]
            tunnel: w402 -> [w441]
            n146 = for {
              tunnel: w442 -> [w451] mode=indexing
              tunnel: [w450] -> w447 mode=indexing
              n147 = Unbundle By Name(w451) -> ("PU"=w450:T7)
            }
            n148 = call "PH_BeamlineInformation.get Head Information by PU.vi"("Heads"=w441, "Power Unit"=w438) -> ("In Use linked?"=w439:bool, "In Use GUI Ref"=w440:refnum<vi>)  [unwired: 12 in, 4 out]
            n149 = Search 1D Array(1D array=w447, element=w438) -> (index of element=w446:i32)  [unwired: 1 in]
            n150 = Index Array(array=w442, index=w446) -> (element=w445:T6)
            n151 = Unbundle By Name(w445) -> ("Ref Volt"=w444:refnum<vi>)
            n152 = Build Array(w444, w440) -> (w443:refnum<vi>[])
            n153 = for {
              tunnel: w439 -> [w454]
              tunnel: w443 -> [w453] mode=indexing
              shift-right: [w452] -> w449
              shift-left: w448 -> [w455]
              n154 = Not A Number/Path/Refnum?(number/path/refnum=w453) -> (NaN/Path/Refnum?=w456:bool)
              n155 = case shown="False" w456 {
                tunnel: w455 -> [w460 w461]
                tunnel: [w459 w461] -> w452
                tunnel: w453 -> [w458 _]
                tunnel: w454 -> [w457 _]
                frame False {
                  n156 = property class="Ctl"(reference=w458, error in=w460, "Visible"=w457) -> (error out=w459:errorcluster)  [unwired: 1 out]
                }
                frame True {
                }
              }
            }
          }
        }
      }
    }
    frame Error {
    }
  }
  "answer cluster" <- w7
  "i ref out" <- w4
  "error out" <- w3
